vi "sv_Fractional-octave Analysis (1 Ch).vi"(0 "scaled signal [EU]":waveform(dbl), 1 "1/n Octave settings":T7={"standard"=enum."ANSI S1.11", "bandwidth"=enum."1/3 octave"}, 5 "band number":cluster{"low band":i32, "high band":i32}, 7 "restart averaging (F)":bool, 9 "reset filter (F)":bool, 11 "error in (no error)":errorcluster, 12 "averaging type":T8(ring)=enum."Exponential", 13 "exp avg settings":T5={" mode"=enum."Fast", "time constant [ms]"=125.0} {"time constant [ms]" format="%.2f"}, 14 "equal confidence level [dB]":dbl=125.0 format="%.2f") -> (3 "settled?":bool, 4 "octave spectrum":T6 {"band power [EU^2 rms]" format="%.2f"; "nominal frequencies [Hz]" format="%.2f"}, 6 "# samples to settle":u64, 10 "octave info":T1={"standard"=enum."ANSI S1.11", "bandwidth"=enum."1 octave", "low band"=0, "high band"=0, "weighting filter"=0, "dB reference"=0.0, "dB On"=FALSE, "unit label"="", "channel name"="", "description"="", "engineering units"=1, "custom label"="", "spectrum type"=enum."magnitude", "spectral density"=FALSE, "filters settled"=FALSE} {"engineering units" items=["custom..."=0, "V"=1, "A"=21, "C"=30, "pC"=31, "s"=32, "-"=29, "Pa"=2, "N"=20, "g"=3, "m/s^2"=4, "m/s"=5, "m"=6, "mm/s"=12, "mm"=13, "micron/s"=14, "micron"=15, "in/s^2"=7, "in/s"=8, "in"=9, "mil/s"=10, "mil"=11, "rad/s^2"=16, "rad/s"=17, "rad"=18, "deg/s^2"=26, "deg/s"=27, "deg"=28, "RPM"=22, "cycle/s^2"=23, "Hz"=24, "cycle"=25, "strain"=19]; "dB reference" format="%.2e"; "weighting filter" items=["Linear", "A-weighting", "B-weighting", "C-weighting", "ITU-R 468-4", "Dolby", "CCITT", "C-message", "Wb", "Wc", "Wd", "We", "Wf", "Wh", "Wj", "Wk", "Wm", "AES17 20 kHz lowpass", "AES17 40 kHz lowpass", "AES17 20 kHz highpass", "AES17 40 kHz highpass"]}, 15 "error out":errorcluster)   [LabVIEW 2017, in "SoundVib_Octave.lvlib"]
doc: "Performs a fractional-octave analysis on the input signal.\nThe fractional-octave filters are designed in accordance with one of the following standards:\n ANSI S1.11-1986, Order 3, Type 1-D, optional range;\n Fractional-octave-band filters, class 1, IEC 1260:1995.\nFor both standards, the sampling frequency must be at least 3 times the highest midband frequency for octave analysis and at least 2.5 times the highest midband frequency for 1/3, 1/6, 1/12, or 1/24 octave analysis. Available bandwidths are 1/1, 1/3, 1/6, 1/12, and 1/24 octave.\nThe frequency range is based on the low and high bands specified in the band number cluster. A value of 0 corresponds to the reference frequency of the audio-frequency \nrange 1 kHz. Each successive value corresponds to the next fractional-octave band. Positive values cover the range above 1 kHz, and negative values cover the range below 1 kHz.\nAvailable averaging types are Linear, Exponential (default), Equal confidence, and Peak. Based on the selected averaging type, this VI uses the additional settings in averaging parameters.\nThis VI returns the power in each fractional-octave band.\nTo ensure a continuous filtering operation call this VI the first time with filter init/cont set to FALSE and then call it with filter init/cont set to TRUE."
uses:
  <vilib>/addons/Sound and Vibration/svt_Octave/SoundVib_Octave.lvlib
  <vilib>/addons/_NISVFA/_Shared subVIs/Controls/svc_Octave Standard.ctl
  <vilib>/addons/_NISVFA/_Shared subVIs/Controls/svc_Octave Info.ctl
  <vilib>/addons/_NISVFA/_Shared subVIs/Controls/svc_Weighting Filter Text Ring.ctl
  <vilib>/addons/_NISVFA/_Shared subVIs/Controls/svc_Engineering Units Text Ring.ctl
  <vilib>/addons/Sound and Vibration/svt_Octave_2014 standard/SoundVib_Octave_2014 standard.lvlib
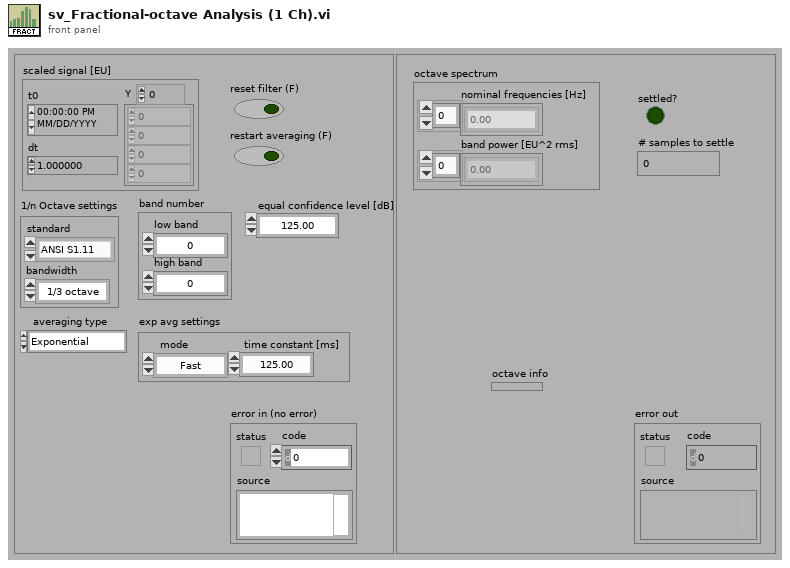
[diagram p1: front panel]
types:
  T1 = typedef "svc_Octave Info.ctl" = cluster{"standard":T2, "bandwidth":enum16{"1 octave", "1/3 octave", "1/6 octave", "1/12 octave", "1/24 octave"}, "low band":i32, "high band":i32, "weighting filter":T3, "dB reference":dbl, "dB On":bool, "unit label":string, "channel name":string, "description":string, "engineering units":T4, "custom label":string, "spectrum type":enum16{"power", "magnitude"}, "spectral density":bool, "filters settled":bool}
  T2 = typedef "svc_Octave Standard.ctl" = enum16{"ANSI S1.11", "IEC 61260"}
  T3 = typedef "svc_Weighting Filter Text Ring.ctl" = u16
  T4 = typedef "svc_Engineering Units Text Ring.ctl" = u16
  T5 = cluster{" mode":enum16{"Slow", "Fast", "Impulse", "Custom"}, "time constant [ms]":dbl}
  T6 = cluster{"nominal frequencies [Hz]":dbl[], "band power [EU^2 rms]":dbl[]}
  T7 = cluster{"standard":T2, "bandwidth":enum16{"1 octave", "1/3 octave", "1/6 octave", "1/12 octave", "1/24 octave"}}
  T8 = enum16{"Linear", "Exponential", "Equal confidence", "Peak"}
  T9 = enum16{"1 octave", "1/3 octave", "1/6 octave", "1/12 octave", "1/24 octave", "1/48 octave", "1/96 octave"}
  T10 = cluster{"# special filters":i32, "special filter coefficients":cluster{"filter structure":enum32{"IIR 2nd Order", "IIR 4th Order"}, "Reverse Coefficients":dbl[], "Forward Coefficients":dbl[]}[], "# filters per octave":cluster{"# filters":i32, "starting at":i32}[], "standard filter coefficients":cluster{"filter structure":enum32{"IIR 2nd Order", "IIR 4th Order"}, "Reverse Coefficients":dbl[], "Forward Coefficients":dbl[]}[], "# decimation steps":i32, "lowpass filter coefficients":cluster{"filter structure":enum32{"IIR 2nd Order", "IIR 4th Order"}, "Reverse Coefficients":dbl[], "Forward Coefficients":dbl[]}, "# samples to settle":u64, "special filter bandwidth":dbl[], "standard filter bandwidth":dbl[]}
  T11 = cluster{"octave filter":cluster{"Octave filter":dbl[]}[], "decimation":i32[], "lowpass filter":dbl[][], "exponential averaging":cluster{"exponential averaging":dbl, "peak detector":dbl}[], "linear averaging":cluster{"squared sum":dbl, "size":dbl}[], "result":dbl[], "# samples since init":u64}
  T12 = enum16{"1 octave", "1/3 octave", "1/6 octave", "1/12 octave", "1/24 octave"}
  T13 = cluster{"dup nominal frequencies [Hz":dbl[], "band power [EU^2 rms]":dbl[]}
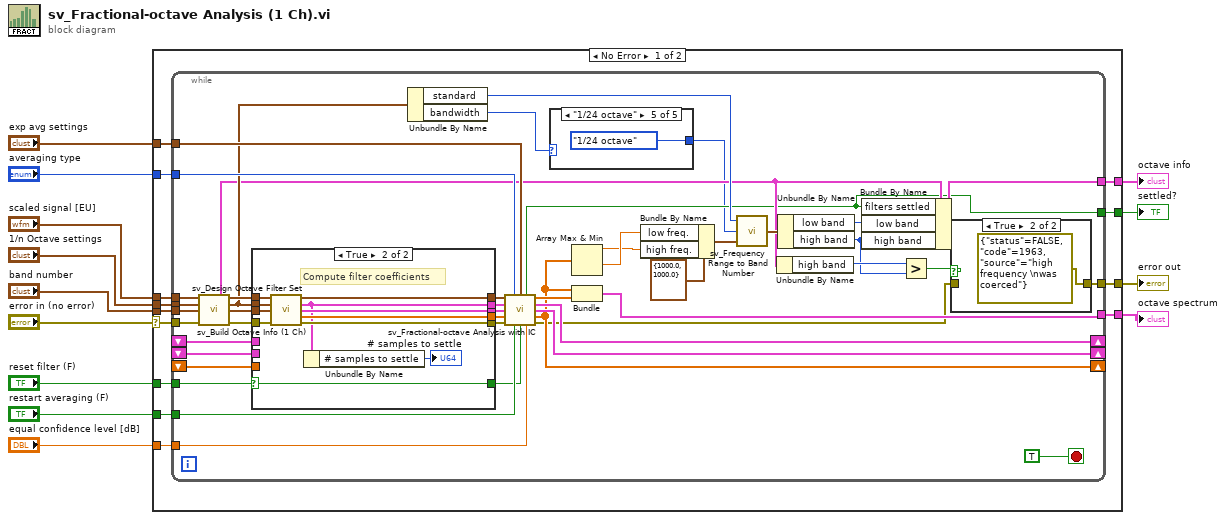
[diagram p0: block diagram]
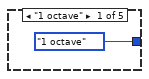
[diagram p2: hidden frame]
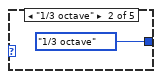
[diagram p3: hidden frame]
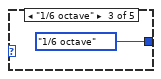
[diagram p4: hidden frame]
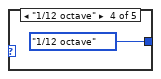
[diagram p5: hidden frame]
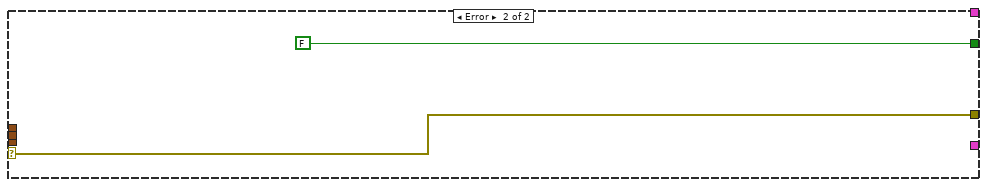
[diagram p8: hidden frame]
diagram:
  n1 = case shown="No Error" "error in (no error)" {
    selector: "error in (no error)" -> [w15 w96]
    tunnel: "reset filter (F)" -> [w26 _]
    tunnel: "scaled signal [EU]" -> [w25 _]
    tunnel: "band number" -> [w24 _]
    tunnel: "restart averaging (F)" -> [w23 _]
    tunnel: "averaging type" -> [w22 _]
    tunnel: [w21 w96] -> w8
    tunnel: "1/n Octave settings" -> [w20 _]
    tunnel: [w19 FALSE ("filter settled ?")] -> w6
    tunnel: [w14 _] -> w5
    tunnel: "exp avg settings" -> [w18 _]
    tunnel: "equal confidence level [dB]" -> [w17 _]
    tunnel: [w16 _] -> w2
    frame No Error {
      n2 = while {
        tunnel: [w40] -> w16
        tunnel: w17 -> [w56]
        tunnel: w18 -> [w57]
        tunnel: [w32] -> w21
        tunnel: w15 -> [w55]
        tunnel: [w31] -> w19
        tunnel: w20 -> [w52]
        tunnel: w22 -> [w65]
        tunnel: w23 -> [w66]
        tunnel: w24 -> [w53]
        tunnel: w25 -> [w54]
        tunnel: w26 -> [w67]
        shift-left: _ -> [w69]
        shift-right: [w46] -> _
        shift-left: _ -> [w71]
        shift-right: [w61] -> _
        shift-left: _ -> [w70]
        shift-right: [w58] -> _
        tunnel: [w45] -> w14
        stop <- TRUE stop-if-true
        n3 = call <vilib>:"sv_Build Octave Info (1 Ch).vi"("scaled signal [EU]"=w54, "1/n octave settings"=w52, "band number"=w53, "error in (no error)"=w55) -> ("octave info"=w37:T1, "dup scaled signal [EU]"=w49:waveform(dbl), "dup 1/n octave settings"=w41:T7, "dup band number"=w51:cluster{"low band":i32, "high band":i32}, "error out"=w50:errorcluster)  [unwired: 7 in]
        n4 = case shown="True" w67 {
          selector: w67 -> [w83 w95]
          tunnel: [w84 w88] -> w62
          tunnel: w71 -> [w82 _]
          tunnel: w70 -> [w84 _]
          tunnel: w69 -> [w80 _]
          tunnel: [w83 w95] -> w48
          tunnel: w49 -> [w81 w91]
          tunnel: [w82 w86] -> w63
          tunnel: [w81 w92] -> w64
          tunnel: [w79 w93] -> w60
          tunnel: [w80 w87] -> w59
          tunnel: w41 -> [_ w90]
          tunnel: w51 -> [_ w89]
          tunnel: w50 -> [w79 w94]
          frame False {
            # "Use previously calculated coefficients"
          }
          frame True {
            # "Compute filter coefficients"
            n5 = call <vilib>:"sv_Design Octave Filter Set.vi"("scaled signal [EU]"=w91, "1/n octave settings"=w90, "band number"=w89, "error in (no error)"=w94) -> ("dup scaled signal [EU]"=w92:waveform(dbl), "filter bank parameters"=w86:T10, "initial filter state"=w88:T11, "nominal frequencies [Hz]"=w87:dbl[], "error out"=w93:errorcluster)  [unwired: 7 in]
            n6 = Unbundle By Name(w86) -> ("# samples to settle"=→"# samples to settle":u64)
          }
        }
        n7 = Unbundle By Name(w41) -> ("standard"=w42:T2, "bandwidth"=w28:T12)
        n8 = call <vilib>:"sv_Fractional-octave Analysis with IC.vi"("scaled signal [EU]"=w64, "averaging type"=w65, "exp avg settings"=w57, "filter bank parameters"=w63, "internal filter state IN"=w62, "nominal frequencies [Hz]"=w59, "error in (no error)"=w60, "restart averaging (F)"=w66, "reset filter"=w48, "equal confidence level [dB]"=w56) -> ("filter settled ?"=w31:bool, "band power [EU^2 rms]"=w47:dbl[], "dup filter bank parameters"=w61:T10, "internal filter state OUT"=w58:T11, "dup nominal frequencies [Hz"=w46:dbl[], "error out"=w33:errorcluster)
        n9 = case shown="\"1/24 octave\"" w28 {
          tunnel: [T9."1 octave" ("bandwidth") T9."1/3 octave" ("bandwidth") T9."1/6 octave" ("bandwidth") T9."1/12 octave" ("bandwidth") T9."1/24 octave" ("bandwidth")] -> w27
          frame "1 octave" {
          }
          frame "1/3 octave" {
          }
          frame "1/6 octave" {
          }
          frame "1/12 octave" {
          }
          frame "1/24 octave" {
          }
        }
        n10 = Array Max & Min(array=w46) -> (max value=w43:dbl, min value=w44:dbl)  [unwired: 2 out]
        n11 = Bundle("dup nominal frequencies [Hz"=w46, "band power [EU^2 rms]"=w47) -> (w45:T13)  [unwired: 1 in]
        n12 = Bundle By Name(cluster=cluster{"low freq.":dbl, "high freq.":dbl} {"low freq."=1000.0, "high freq."=1000.0} ("frequency range [Hz]"), "low freq."=w44, "high freq."=w43) -> (w30:cluster{"low freq.":dbl, "high freq.":dbl})
        n13 = call <vilib>:"sv_Frequency Range to Band Number.vi"("frequency range [Hz]"=w30, "bandwidth"=w27, "standard"=w42) -> ("band number"=w39:cluster{"low band":i32, "high band":i32})
        n14 = Unbundle By Name(w37) -> ("high band"=w36:i32)
        n15 = Unbundle By Name(w39) -> ("low band"=w38:i32, "high band"=w35:i32)
        n16 = Bundle By Name(cluster=w37, "filters settled"=w31, "low band"=w38, "high band"=w35) -> (w40:T1)
        n17 = Greater?(x=w36, y=w35) -> (0:w34:bool)
        n18 = case shown="True" w34 {
          tunnel: w33 -> [w77 _]
          tunnel: [w77 errorcluster {"status"=FALSE, "code"=1963, "source"="high frequency \nwas coerced"} ("error IO")] -> w32
          frame False {
          }
          frame True {
          }
        }
      }
    }
    frame Error {
    }
  }
  "settled?" <- w6
  "error out" <- w8
  "octave spectrum" <- w5
  "octave info" <- w2
